vi "Format.vi"(8 "Error in (no error)":errorcluster, 10 "Log in":T1 {"Priority" items=["EMERGENCY", "ALERT", "CRITICAL", "ERROR", "WARNING", "NOTICE", "INFO", "DEBUG"]}, 11 "LogFormatterInterface in":refnum<class "LogFormatterInterface.lvclass">) -> (0 "Error out":errorcluster, 2 "Log formatted":string, 3 "LogFormatterInterface out":refnum<class "LogFormatterInterface.lvclass">)   [LabVIEW 2011, in "LogFormatterInterface.lvclass"]
uses:
  LogFormatterInterface.lvclass
  Log/LogCluster.ctl
  Log/PrioritiesRing.ctl
  Log/Log.lvclass
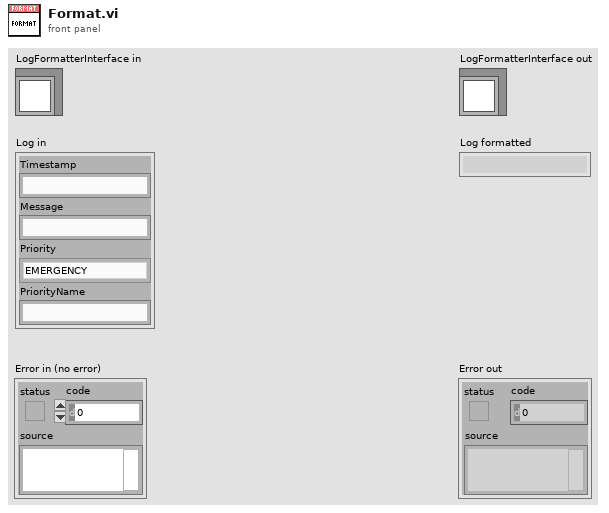
[diagram p1: front panel]
types:
  T1 = typedef "Log.lvclass/LogCluster.ctl" = cluster{"Timestamp":string, "Message":string, "Priority":T2, "PriorityName":string}
  T2 = typedef "Log.lvclass/PrioritiesRing.ctl" = u32
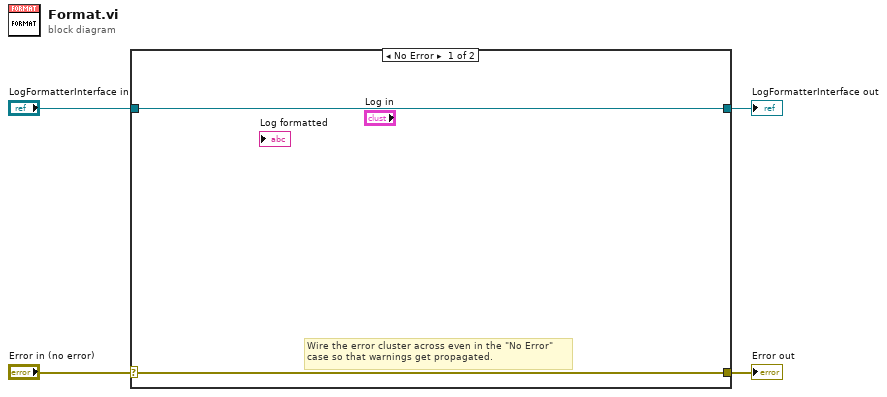
[diagram p0: block diagram]
diagram:
  n1 = case shown="No Error" "Error in (no error)" {
    selector: "Error in (no error)" -> [w5 w8]
    tunnel: [w5 w8] -> w3
    tunnel: [w6 w7] -> w1
    tunnel: "LogFormatterInterface in" -> [w6 w7]
    frame No Error {
      # "Wire the error cluster across even in the \"No Error\"\ncase so that warnings get propagated."
    }
    frame Error {
    }
  }
  "Error out" <- w3
  "LogFormatterInterface out" <- w1
